vi "Ball System.vi"(0 "Ball System Actions":T1) -> ()   [LabVIEW 2019]
uses:
  Controls/Ball System Actions.ctl
  <vilib>/Rock Robotics/Network Tables/NT Read Number.vi
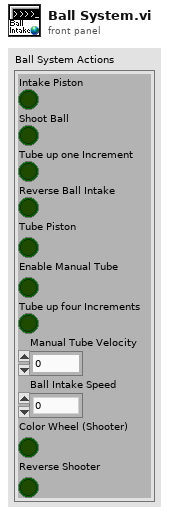
[diagram p1: front panel]
types:
  T1 = typedef "Ball System Actions.ctl" = cluster{"Intake Piston ":bool, "Shoot Ball":bool, "Tube up one Increment\t":bool, "Reverse Ball Intake":bool, "Tube Piston":bool, "Enable Manual Tube":bool, "Tube up four Increments":bool, "Manual Tube Velocity":dbl, "Ball Intake Speed":dbl, "Color Wheel (Shooter)":bool, "Reverse Shooter":bool}
  T2 = typedef "WPI_MotorControlDeviceRef.ctl" = cluster{"DeviceStatus":errorcluster, "Type":T3, "PWM":cluster{"PWM Channel":T4, "DeadBand":T5}, "CAN":cluster{"Device Number":u8, "SetOutput VI Ref":variant, "GetOutput VI Ref":variant, "Enable VI Ref":variant, "Disable VI Ref":variant, "Data":variant}, "Invert":bool, "DIO PWM":cluster{"PWM \"Enable\" Channel":T4, "DIOChannel":T6, "PWM Rate":dbl}}
  T3 = typedef "WPI_MotorControlType.ctl" = enum16{"PWM", "CAN", "DIO PWM"}
  T4 = typedef "FPGA_DIOPWMChannel.ctl" = enum8{"PWM 0", "PWM 1", "PWM 2", "PWM 3", "PWM 4", "PWM 5", "PWM 6", "PWM 7", "PWM 8", "PWM 9", "PWM MXP 0", "PWM MXP 1", "PWM MXP 2", "PWM MXP 3", "PWM MXP 4", "PWM MXP 5", "PWM MXP 6", "PWM MXP 7", "PWM MXP 8", "PWM MXP 9", "Invalid"}
  T5 = typedef "WPI_PWMDeadband.ctl" = cluster{"Name":string, "maxPositivePwm":i32, "minPositivePwm":i32, "centerPwm":i32, "maxNegativePwm":i32, "minNegativePwm":i32, "angularRange":u16}
  T6 = typedef "FPGA_DIOChannel.ctl" = enum8{"DIO 0", "DIO 1", "DIO 2", "DIO 3", "DIO 4", "DIO 5", "DIO 6", "DIO 7", "DIO 8", "DIO 9", "DIO MXP 0", "DIO MXP 1", "DIO MXP 2", "DIO MXP 3", "DIO MXP 4", "DIO MXP 5", "DIO MXP 6", "DIO MXP 7", "DIO MXP 8", "DIO MXP 9", "DIO MXP 10", "DIO MXP 11", "DIO MXP 12", "DIO MXP 13", "DIO MXP 14", "DIO MXP 15", "SPI Port CS1", "SPI Port CS2", "SPI Port CS3", "SPI Port MISO", "SPI Port MOSI", "Invalid"}
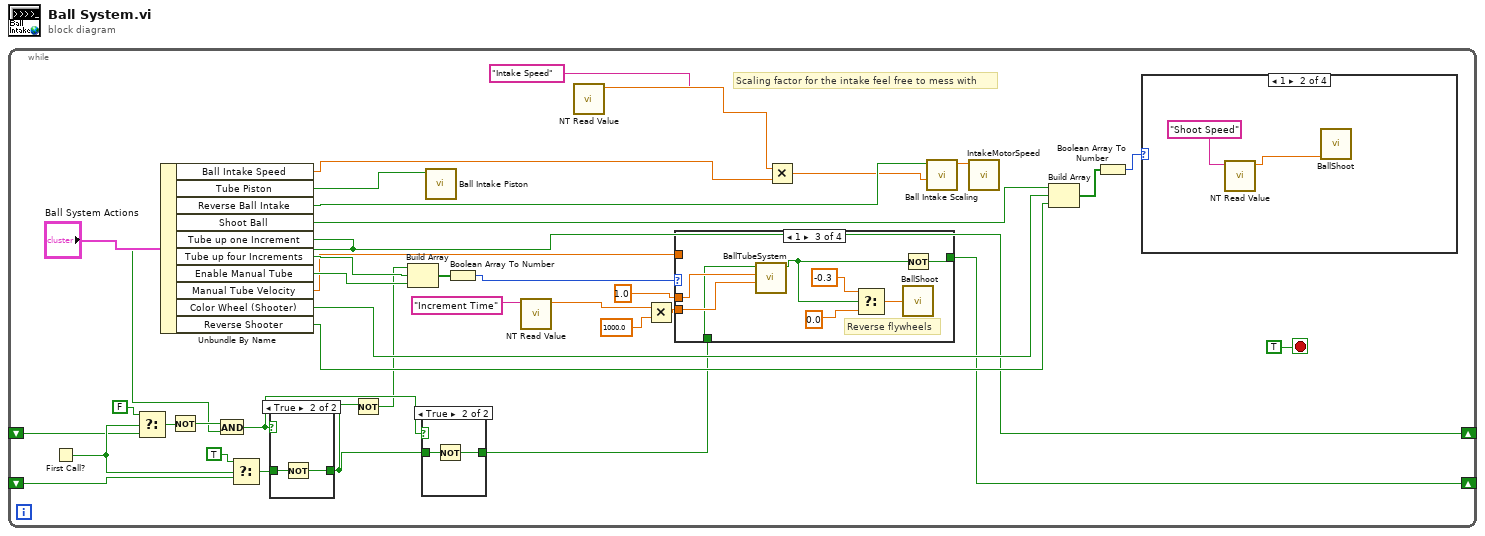
[diagram p0: block diagram]
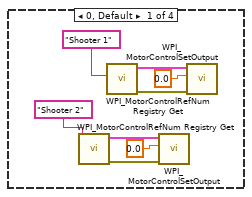
[diagram p4: hidden frame]
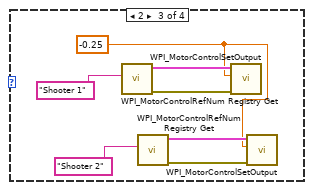
[diagram p5: hidden frame]
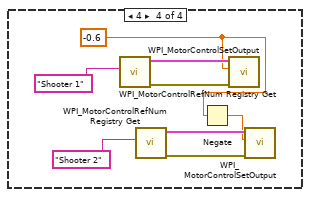
[diagram p6: hidden frame]
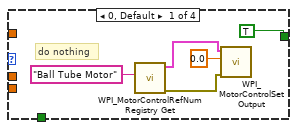
[diagram p7: hidden frame]
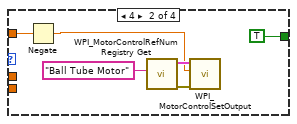
[diagram p8: hidden frame]
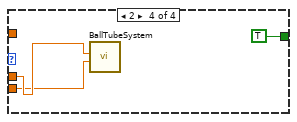
[diagram p9: hidden frame]
diagram:
  n1 = while {
    shift-right: [w12] -> _
    shift-left: _ -> [w11]
    shift-right: [w10] -> _
    shift-left: _ -> [w9]
    stop <- TRUE stop-if-true
    # "Scaling factor for the intake feel free to mess with"
    n2 = First Call?() -> (First Call?: T/F=w16:bool)
    n3 = Select(t=FALSE, s=w16, f=w11) -> (s? t:f=w14:bool)
    n4 = Unbundle By Name("Ball System Actions") -> ("Ball Intake Speed"=w27:dbl, "Tube Piston"=w30:bool, "Reverse Ball Intake"=w29:bool, "Shoot Ball"=w25:bool, "Tube up one Increment"=w12:bool, "Tube up four Increments"=w36:bool, "Enable Manual Tube"=w35:bool, "Manual Tube Velocity"=w32:dbl, "Color Wheel (Shooter)"=w24:bool, "Reverse Shooter"=w21:bool)
    n5 = Not(x=w14) -> (.not. x?=w18:bool)
    n6 = And(x=w18, y=w12) -> (x .and. y?=w4:bool)
    n7 = Select(t=TRUE, s=w16, f=w9) -> (s? t:f=w13:bool)
    n8 = case shown="True" w4 {
      tunnel: [w42 w44] -> w2
      tunnel: w13 -> [w42 w43]
      frame False {
      }
      frame True {
        n9 = Not(x=w43) -> (.not. x?=w44:bool)
      }
    }
    n10 = Not(x=w2) -> (.not. x?=w1:bool)
    n11 = Build Array(w1, w36, w35) -> (w33:bool[])
    n12 = case shown="True" w4 {
      tunnel: w2 -> [w39 w41]
      tunnel: [w39 w40] -> w3
      frame False {
      }
      frame True {
        n13 = Not(x=w41) -> (.not. x?=w40:bool)
      }
    }
    n14 = call "Ball Intake Piston.vi"("Tube Piston"=w30) -> ()  [unwired: 11 in]
    n15 = Boolean Array To Number(Boolean array=w33) -> (number=w38:u32)
    n16 = call-poly <vilib>:"NT Read Value.vi"("Name"="Increment Time") -> ("Numeric"=w7:dbl)  [unwired: 9 in, 1 out]
    n17 = call-poly <vilib>:"NT Read Value.vi"("Name"="Intake Speed") -> ("Numeric"=w20:dbl)  [unwired: 9 in, 1 out]
    n18 = Multiply(x=w7, y=1000.0) -> (x*y=w6:dbl)
    n19 = case shown="1" w38 {
      tunnel: [TRUE TRUE w86 TRUE] -> w10
      tunnel: w32 -> [_ w76 _ _]
      tunnel: 1.0 ("Tube Speed") -> [_ _ w88 w91]
      tunnel: w6 -> [_ _ w87 w90]
      tunnel: w3 -> [_ _ w85 _]
      frame 0, Default {
        # "do nothing"
        n20 = call <vilib>:"WPI_MotorControlRefNum Registry Get.vi"("refnum name"="Ball Tube Motor") -> ("error out"=w74:errorcluster, "MotorControlDevRef"=w73:T2)  [unwired: 9 in]
        n21 = call <vilib>:"WPI_MotorControlSetOutput.vi"("error in (no error)"=w74, "Output"=0.0, "MotorControlDevRef"=w73) -> ()  [unwired: 6 in, 3 out]
      }
      frame 4 {
        n22 = Negate(x=w76) -> (-x=w75:dbl)
        n23 = call <vilib>:"WPI_MotorControlRefNum Registry Get.vi"("refnum name"="Ball Tube Motor") -> ("error out"=w80:errorcluster, "MotorControlDevRef"=w79:T2)  [unwired: 9 in]
        n24 = call <vilib>:"WPI_MotorControlSetOutput.vi"("error in (no error)"=w80, "Output"=w75, "MotorControlDevRef"=w79) -> ()  [unwired: 6 in, 3 out]
      }
      frame 1 {
        # "Reverse flywheels"
        n25 = call "BallTubeSystem.vi"("Duration in ms"=w87, "Tube Speed"=w88, "Initialize"=w85) -> ("Running"=w84:bool)  [unwired: 6 in, 1 out]
        n26 = Select(t=-0.3, s=w84, f=0.0) -> (s? t:f=w83:dbl)
        n27 = Not(x=w84) -> (.not. x?=w86:bool)
        n28 = call "BallShoot.vi"("Scaling"=w83) -> ()  [unwired: 11 in]
      }
      frame 2 {
        n29 = call "BallTubeSystem.vi"("Duration in ms"=w90, "Tube Speed"=w91) -> ()  [unwired: 7 in, 2 out]
      }
    }
    n30 = Multiply(x=w20, y=w27) -> (x*y=w26:dbl)
    n31 = call "Ball Intake Scaling.vi"("Scaling factor"=w26, "Intake"=w29) -> ("IntakeSpeed"=w31:dbl)  [unwired: 9 in]
    n32 = call "IntakeMotorSpeed.vi"("IntakeSpeed"=w31) -> ()  [unwired: 11 in]
    n33 = Build Array(w25, w24, w21) -> (w23:bool[])
    n34 = Boolean Array To Number(Boolean array=w23) -> (number=w22:u32)
    n35 = case shown="1" w22 {
      frame 0, Default {
        n36 = call <vilib>:"WPI_MotorControlRefNum Registry Get.vi"("refnum name"="Shooter 2") -> ("error out"=w47:errorcluster, "MotorControlDevRef"=w46:T2)  [unwired: 9 in]
        n37 = call <vilib>:"WPI_MotorControlRefNum Registry Get.vi"("refnum name"="Shooter 1") -> ("error out"=w50:errorcluster, "MotorControlDevRef"=w51:T2)  [unwired: 9 in]
        n38 = call <vilib>:"WPI_MotorControlSetOutput.vi"("error in (no error)"=w47, "Output"=0.0, "MotorControlDevRef"=w46) -> ()  [unwired: 6 in, 3 out]
        n39 = call <vilib>:"WPI_MotorControlSetOutput.vi"("error in (no error)"=w50, "Output"=0.0, "MotorControlDevRef"=w51) -> ()  [unwired: 6 in, 3 out]
      }
      frame 1 {
        n40 = call-poly <vilib>:"NT Read Value.vi"("Name"="Shoot Speed") -> ("Numeric"=w54:dbl)  [unwired: 9 in, 1 out]
        n41 = call "BallShoot.vi"("Scaling"=w54) -> ()  [unwired: 11 in]
      }
      frame 2 {
        w55 = -0.25 ("y")
        n42 = call <vilib>:"WPI_MotorControlRefNum Registry Get.vi"("refnum name"="Shooter 1") -> ("error out"=w60:errorcluster, "MotorControlDevRef"=w61:T2)  [unwired: 9 in]
        n43 = call <vilib>:"WPI_MotorControlRefNum Registry Get.vi"("refnum name"="Shooter 2") -> ("error out"=w57:errorcluster, "MotorControlDevRef"=w56:T2)  [unwired: 9 in]
        n44 = call <vilib>:"WPI_MotorControlSetOutput.vi"("error in (no error)"=w60, "Output"=w55, "MotorControlDevRef"=w61) -> ()  [unwired: 6 in, 3 out]
        n45 = call <vilib>:"WPI_MotorControlSetOutput.vi"("error in (no error)"=w57, "Output"=w55, "MotorControlDevRef"=w56) -> ()  [unwired: 6 in, 3 out]
      }
      frame 4 {
        w63 = -0.6 ("y")
        n46 = call <vilib>:"WPI_MotorControlRefNum Registry Get.vi"("refnum name"="Shooter 1") -> ("error out"=w68:errorcluster, "MotorControlDevRef"=w69:T2)  [unwired: 9 in]
        n47 = call <vilib>:"WPI_MotorControlRefNum Registry Get.vi"("refnum name"="Shooter 2") -> ("error out"=w65:errorcluster, "MotorControlDevRef"=w64:T2)  [unwired: 9 in]
        n48 = Negate(x=w63) -> (-x=w62:dbl)
        n49 = call <vilib>:"WPI_MotorControlSetOutput.vi"("error in (no error)"=w68, "Output"=w63, "MotorControlDevRef"=w69) -> ()  [unwired: 6 in, 3 out]
        n50 = call <vilib>:"WPI_MotorControlSetOutput.vi"("error in (no error)"=w65, "Output"=w62, "MotorControlDevRef"=w64) -> ()  [unwired: 6 in, 3 out]
      }
    }
  }
